vi "arm-sim-globals.vi"() -> ()   [LabVIEW 2020]
panel:
  out "arm-sim-lift-pos-raw":dbl
  out "arm-sim-ext-pos-raw":dbl
  out "arm-sim-ext-atlowlimit":bool
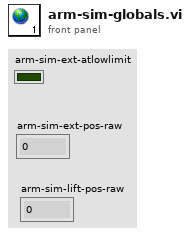
[diagram p1: front panel]
diagram:
